vi "initClass_View.vi"(8 "error in (no error)":errorcluster, 9 "TypeFirmware":T1, 10 "Queue Process":T2, 11 "XuLyDataDisplay in":refnum<class "XuLyDataDisplay.lvclass">) -> (0 "error out":errorcluster, 3 "XuLyDataDisplay out":refnum<class "XuLyDataDisplay.lvclass">)   [LabVIEW 2017, in "LibraryGcode.lvlib" / "XuLyDataDisplay.lvclass"]
uses:
  XuLyDataDisplay.lvclass
  control/Queue/QueueCMDandPOS.ctl
  control/Queue/TypeDataPOS.ctl
  control/stateCmdUpdatePara.ctl
  control/TypeFirmwareControl.ctl
  ClassParameter/stateLoop_View.ctl
  ClassParameter/ParameterConf.lvclass
  LibraryGcode.lvlib
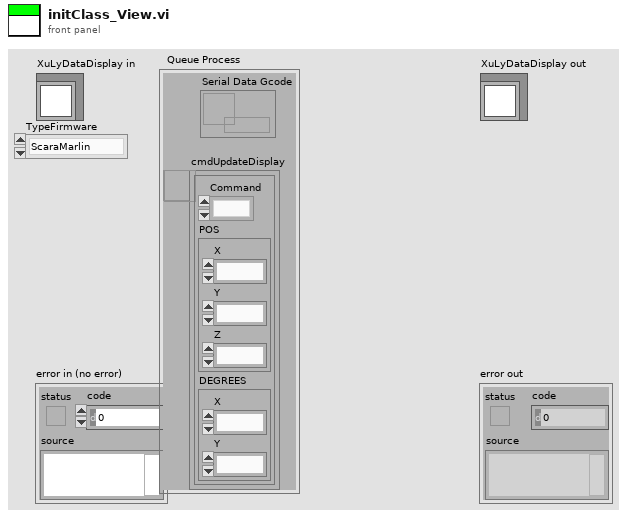
[diagram p1: front panel]
types:
  T1 = typedef "LibraryGcode.lvlib/TypeFirmwareControl.ctl" = enum16{"ScaraMarlin", "CncMarlin", "Mk4Due"}
  T2 = typedef "LibraryGcode.lvlib/QueueCMDandPOS.ctl" = cluster{"Serial Data Gcode":refnum<queue>, "cmdUpdateDisplay":refnum<queue>}
  T3 = typedef "LibraryGcode.lvlib/ParameterConf.lvclass/stateLoop_View.ctl" = enum16{"Running", "writeGlobal", "schedules500ms", "init", "End"}
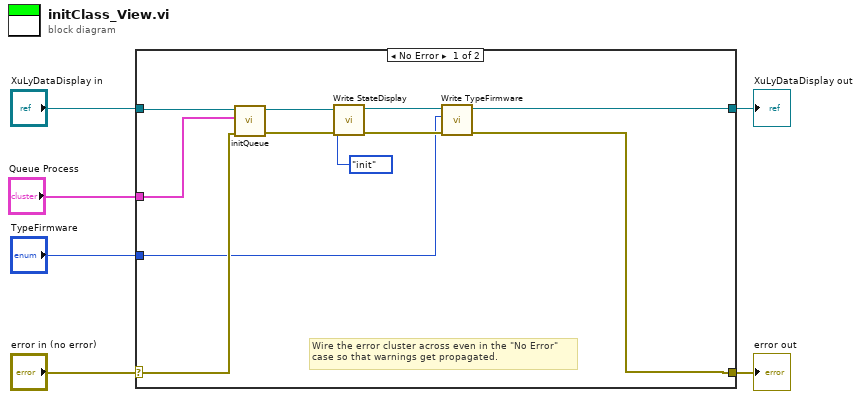
[diagram p0: block diagram]
diagram:
  n1 = case shown="No Error" "error in (no error)" {
    selector: "error in (no error)" -> [w15 w19]
    tunnel: [w10 w19] -> w5
    tunnel: [w11 w18] -> w3
    tunnel: "XuLyDataDisplay in" -> [w17 w18]
    tunnel: "Queue Process" -> [w13 _]
    tunnel: "TypeFirmware" -> [w8 _]
    frame No Error {
      # "Wire the error cluster across even in the \"No Error\"\ncase so that warnings get propagated."
      n2 = call-dynamic "initQueue.vi"("error in (no error)"=w15, "Queue Process"=w13, "ParameterConf in"=w17) -> ("error out"=w14:errorcluster, "ParameterConf out"=w16:refnum<class "XuLyDataDisplay.lvclass">)  [unwired: 7 in]
      n3 = call-dynamic "Write StateDisplay.vi"("error in (no error)"=w14, "StateDisplay"=stateLoop_View."init", "ParameterConf in"=w16) -> ("error out"=w9:errorcluster, "ParameterConf out"=w12:refnum<class "XuLyDataDisplay.lvclass">)  [unwired: 7 in]
      n4 = call-dynamic "Write TypeFirmware.vi"("error in (no error)"=w9, "TypeFirmware"=w8, "ParameterConf in"=w12) -> ("error out"=w10:errorcluster, "ParameterConf out"=w11:refnum<class "XuLyDataDisplay.lvclass">)  [unwired: 7 in]
    }
    frame Error {
    }
  }
  "error out" <- w5
  "XuLyDataDisplay out" <- w3
